vi "PAN_run.vi"() -> ()   [LabVIEW 2016]
uses:
  Modules/DBSHAND/private/vis/DatabaseHand_Element_Get(string).vi
panel:
  out "status out":string
  out "mesasage 2":string
  in  "close":bool=TRUE
  # "Pixel  Acquisition Node"
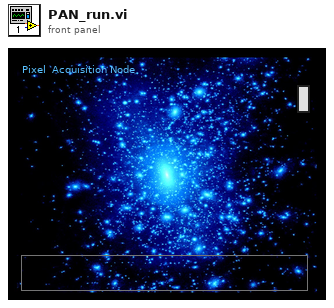
[diagram p1: front panel]
types:
  T1 = enum32{"Invalid", "Standard", "Closed", "Hidden", "Minimized", "Maximized"}
  T2 = typedef "DatabaseHand_RefNum.ctl" = refnum<vi>
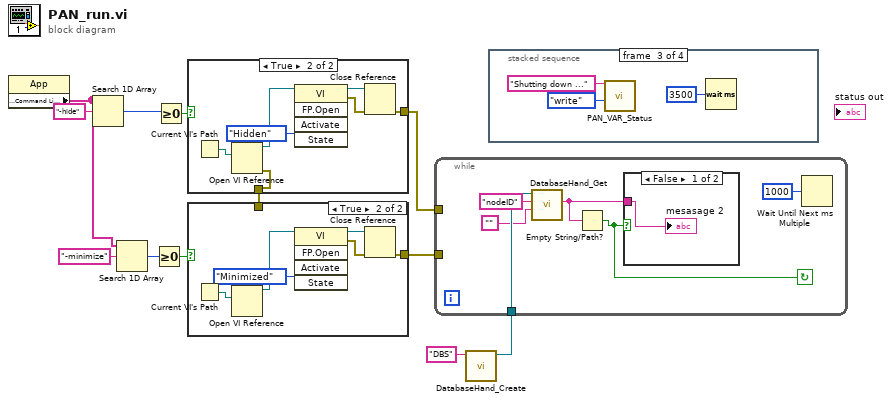
[diagram p0: block diagram]
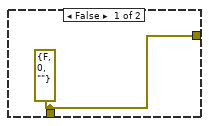
[diagram p4: hidden frame]
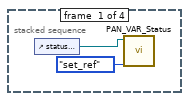
[diagram p5: hidden frame]
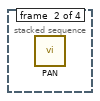
[diagram p6: hidden frame]
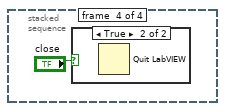
[diagram p7: hidden frame]
diagram:
  n1 = property class="App"() -> ("Application:Command Line Arguments"=w8:string[])  [unwired: 2 in, 2 out]
  n2 = Search 1D Array(1D array=w8, element="-hide") -> (index of element=w11:i32)  [unwired: 1 out]
  n3 = Search 1D Array(1D array=w8, element="-minimize") -> (index of element=w6:i32)  [unwired: 1 out]
  n4 = Greater Or Equal To 0?(x=w6) -> (x >= 0?=w5:bool)
  n5 = Greater Or Equal To 0?(x=w11) -> (x >= 0?=w10:bool)
  n6 = case shown="True" w10 {
    tunnel: [w13 w15] -> w7
    tunnel: [w13 w14] -> w1
    frame False {
      w13 = errorcluster {"status"=FALSE, "code"=0, "source"=""} ("error out")
    }
    frame True {
      n7 = Current VI's Path() -> (path=w20:path)
      n8 = Open VI Reference(vi path=w20) -> (vi reference=w19:refnum<vi>, error out=w15:errorcluster)  [unwired: 1 in, 4 out]
      n9 = invoke class="VI" method="FP.Open"(reference=w19, "State"=T1."Hidden") -> (reference out=w16:refnum<vi>, error out=w17:errorcluster)  [unwired: 3 in, 3 out]
      n10 = Close Reference(reference=w16, error in (no error)=w17) -> (error out=w14:errorcluster)
    }
  }
  n11 = case shown="True" w5 {
    tunnel: w7 -> [w21 _]
    tunnel: [w21 w22] -> w2
    frame False {
    }
    frame True {
      n12 = Current VI's Path() -> (path=w27:path)
      n13 = Open VI Reference(vi path=w27) -> (vi reference=w26:refnum<vi>)  [unwired: 1 in, 5 out]
      n14 = invoke class="VI" method="FP.Open"(reference=w26, "State"=T1."Minimized") -> (reference out=w23:refnum<vi>, error out=w24:errorcluster)  [unwired: 3 in, 3 out]
      n15 = Close Reference(reference=w23, error in (no error)=w24) -> (error out=w22:errorcluster)
    }
  }
  n16 = call "DatabaseHand_Create.vi"("Name"="DBS") -> ("Database RefNum out"=w3:T2)  [unwired: 1 in, 9 out]
  n17 = while {
    tunnel: w3 -> [w32]
    tunnel: w2 -> [_]
    tunnel: w1 -> [_]
    stop <- w28 continue-if-true
    n18 = call-poly "DatabaseHand_Get.vi"("default value"="", "name"="nodeID", "Database RefNum in"=w32) -> ("value"=w29:string)  [unwired: 2 in, 6 out]
    n19 = Empty String/Path?(string/path=w29) -> (empty?=w28:bool)
    n20 = case shown="False" w28 {
      tunnel: w29 -> [w34 _]
      frame False {
        "mesasage 2" <- w34
      }
      frame True {
      }
    }
    n21 = Wait Until Next ms Multiple(millisecond multiple=u32 1000) -> ()  [unwired: 1 out]
  }
  n22 = stacked-sequence {
    frame #0 {
      n23 = control-ref of="status out"() -> (w36:refnum<vi>)
      n24 = call "PAN_VAR_Status.vi"("action"=enum16{"read", "write", "set_ref"}."set_ref", "status"=w36) -> ()  [unwired: 2 in, 8 out]
    }
    frame #1 {
      n25 = call "PAN.vi"() -> ()  [unwired: 1 in, 11 out]
    }
    frame #2 {
      n26 = call "PAN_VAR_Status.vi"("action"=enum16{"read", "write", "set_ref"}."write", "status in"="Shutting down ...") -> ()  [unwired: 2 in, 8 out]
      n27 = Wait (ms)(milliseconds to wait=u32 3500) -> ()  [unwired: 1 out]
    }
    frame #3 {
      n28 = case shown="True" "close" {
        frame False {
        }
        frame True {
          n29 = Quit LabVIEW() -> ()  [unwired: 1 out]
        }
      }
    }
  }
